vi "MethodNodeSetCtrlValDemo.vi"() -> ()   [LabVIEW 2012]
panel:
  out "数值输入控件 2":dbl
  in  "停止按钮":bool
  in  "数值输入控件":dbl
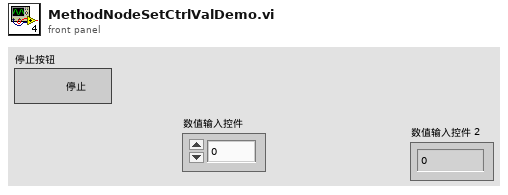
[diagram p1: front panel]
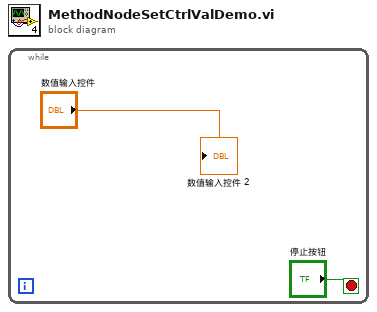
[diagram p0: block diagram]
diagram:
  n1 = while {
    stop <- "停止按钮" stop-if-true
    "数值输入控件 2" <- "数值输入控件"
  }
